vi "Init.vi"(0 "Project Path":path=path "\\\\vmware-host\\Shared Folders/_Repo/DAQ-Waveform-Function-Generator-Custom-Device/Source/Waveform Analog Output Custom Device.lvproj", 5 "Working Directory":path=path "\\\\vmware-host\\Shared Folders/_Repo/DAQ-Waveform-Function-Generator-Custom-Device/Release", 7 "Version":u32=2020, 9 "TCP/IP Port":i32=3363, 11 "error in (no error)":errorcluster) -> (4 "Library Builder out":refnum<class "Library Builder.lvclass">, 15 "error out":errorcluster)   [LabVIEW 2020, in "Library Builder.lvclass"]
uses:
  Library Builder.lvclass
  Library Builder.lvclass/Library Builder.ctl
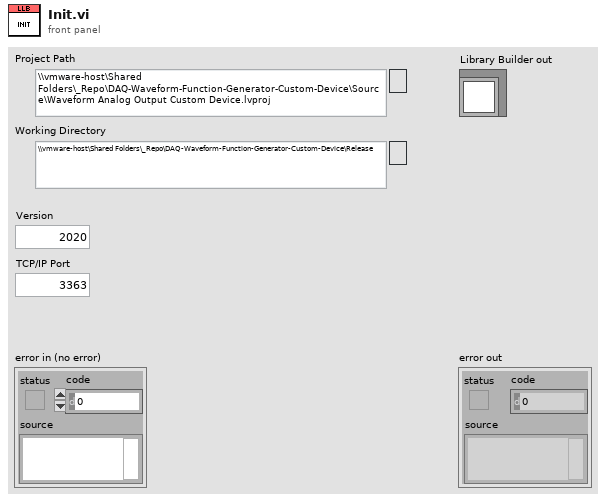
[diagram p1: front panel]
types:
  T1 = enum16{"open", "replace", "create", "open or create", "replace or create", "replace or create with confirmation"}
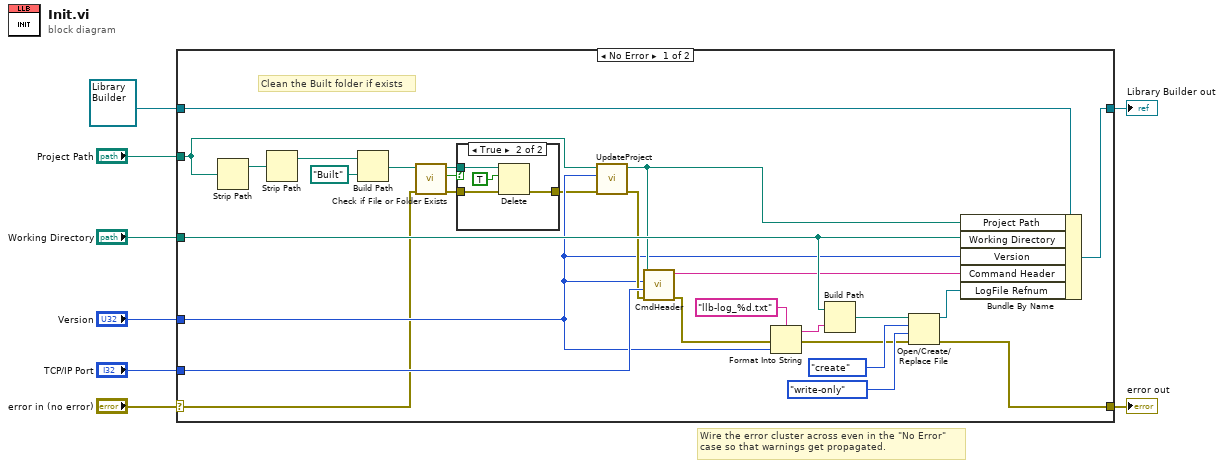
[diagram p0: block diagram]
diagram:
  # "Wire the error cluster across even in the \"No Error\"\ncase so that warnings get propagated."
  n1 = case shown="No Error" "error in (no error)" {
    selector: "error in (no error)" -> [w13 w42]
    tunnel: [w27 w42] -> w7
    tunnel: [w33 w41] -> w6
    tunnel: refnum<class "Library Builder.lvclass"> refnum ("Library Builder in") -> [w34 w41]
    tunnel: "Working Directory" -> [w35 _]
    tunnel: "Project Path" -> [w15 _]
    tunnel: "Version" -> [w19 _]
    tunnel: "TCP/IP Port" -> [w31 _]
    frame No Error {
      # "Clean the Built folder if exists"
      n2 = Strip Path(path=w15) -> (stripped path=w18:path)  [unwired: 1 out]
      n3 = Strip Path(path=w18) -> (stripped path=w17:path)  [unwired: 1 out]
      n4 = Build Path(base path=w17, name or relative path=path "Built") -> (appended path=w14:path)
      n5 = call <vilib>:"Check if File or Folder Exists.vi"("error in (no error)"=w13, "path"=w14) -> ("error out"=w10:errorcluster, "file or folder exists?"=w12:bool, "dup path"=w11:path)  [unwired: 7 in]
      n6 = case shown="True" w12 {
        tunnel: w11 -> [_ w40]
        tunnel: w10 -> [w36 w39]
        tunnel: [w36 w38] -> w9
        frame False {
        }
        frame True {
          n7 = Delete(path (use dialog)=w40, entire hierarchy (F)=TRUE, error in=w39) -> (error out=w38:errorcluster)  [unwired: 2 in, 2 out]
        }
      }
      n8 = call "UpdateProject.vi"("error in (no error)"=w9, "Version"=w19, "Project Path"=w15) -> ("error out"=w21:errorcluster, "Project Path Out"=w20:path)  [unwired: 7 in]
      n9 = call "CmdHeader.vi"("error in (no error)"=w21, "TCP/IP Port"=w31, "Version"=w19, "Project Path"=w20) -> ("error out"=w25:errorcluster, "Command Out"=w32:string)  [unwired: 6 in]
      n10 = Format Into String(format string="llb-log_%d.txt" ("time format string (%c)"), error in=w25, w19) -> (resulting string=w23:string, error out=w24:errorcluster)  [unwired: 1 in]
      n11 = Build Path(base path=w35, name or relative path=w23) -> (appended path=w28:path)
      n12 = Open/Create/Replace File(file path (use dialog)=w28, error in=w24, operation (0:open)=T1."create", access (0:read/write)=enum16{"read/write", "read-only", "write-only"}."write-only") -> (refnum out=w26:refnum<file>, error out=w27:errorcluster)  [unwired: 2 in, 1 out]
      n13 = Bundle By Name(cluster=w34, "Project Path"=w20, "Working Directory"=w35, "Version"=w19, "Command Header"=w32, "LogFile Refnum"=w26) -> (w33:refnum<class "Library Builder.lvclass">)
    }
    frame Error {
    }
  }
  "error out" <- w7
  "Library Builder out" <- w6
